vi "GetObject.vi"(8 "error in (no error)":errorcluster, 11 "Level in":refnum<class "Level.lvclass">) -> (0 "error out":errorcluster, 2 "3D Object.lvclass":refnum<class "3D Object.lvclass">, 3 "Level out":refnum<class "Level.lvclass">)   [LabVIEW 2015, in "Level.lvclass"]
uses:
  Level.lvclass
  3D Object/3D Object.lvclass
  Level.lvclass/Level.ctl
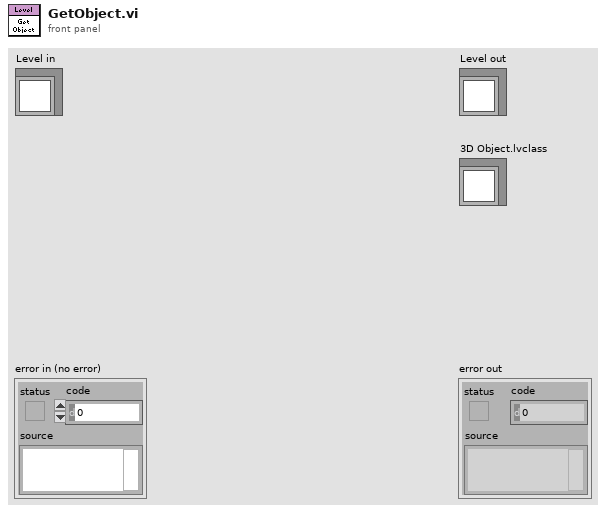
[diagram p1: front panel]
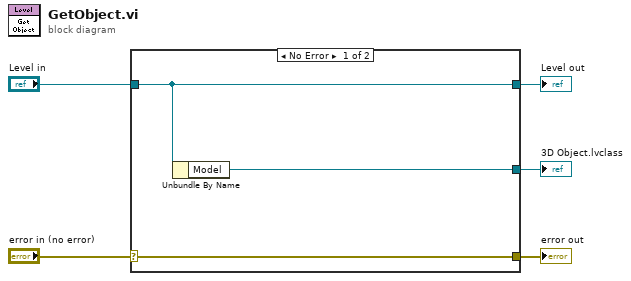
[diagram p0: block diagram]
diagram:
  n1 = case shown="No Error" "error in (no error)" {
    selector: "error in (no error)" -> [w8 w9]
    tunnel: [w8 w9] -> w4
    tunnel: [w7 w10] -> w2
    tunnel: "Level in" -> [w7 w10]
    tunnel: [w6 _] -> w1
    frame No Error {
      n2 = Unbundle By Name(w7) -> ("Model"=w6:refnum<class "3D Object.lvclass">)
    }
    frame Error {
    }
  }
  "error out" <- w4
  "Level out" <- w2
  "3D Object.lvclass" <- w1
